vi "Process Collision.vi"(11 "Ball-Goal Post in":refnum<class "Ball-Goal Post.lvclass">) -> (3 "Ball-Goal Post out":refnum<class "Ball-Goal Post.lvclass">)   [LabVIEW 2021, in "Ball-Goal Post.lvclass"]
doc: "MIT Licence\nCopyright (c) 2024 David Grollier"
uses:
  Ball-Goal Post.lvclass
  C:/Users/David/Documents/GameSoccerSpace/Source/Collision/Collision.lvclass
  Game Componants/Game Board Component/Fixed/Board/Goal post/Goal Post.lvclass
  C:/Users/David/Documents/GameSoccerSpace/Source/Game Componants/Game Componants.lvclass
  Collision.lvclass/Collision.ctl
  Game Componants/Game Board Component/Movable/Movable.lvclass/Movable.ctl
  Game Componants/Game Board Component/Fixed/Board/Goal post/Goal Post.lvclass/Goal Post.ctl
  Game Componants/Game Componants.lvclass/Game Componants.ctl
  <vilib>/Analysis/_algsub.llb/Vector Norm.vi
  <vilib>/Analysis/_algsub.llb/Real Vector Norm.vi
  Game Componants/Game Board Component/Movable/Movable.lvclass
  C:/Users/David/Documents/GameSoccerSpace/Source/Game Componants/Game Board Component/Game Board Component.lvclass
  Collision.lvclass
  Game Componants/Game Componants.lvclass
  Utils/Utils.lvlib
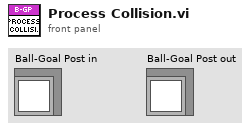
[diagram p1: front panel]
types:
  T1 = typedef "Coordinates.ctl" = cluster{"x":dbl, "y":dbl}
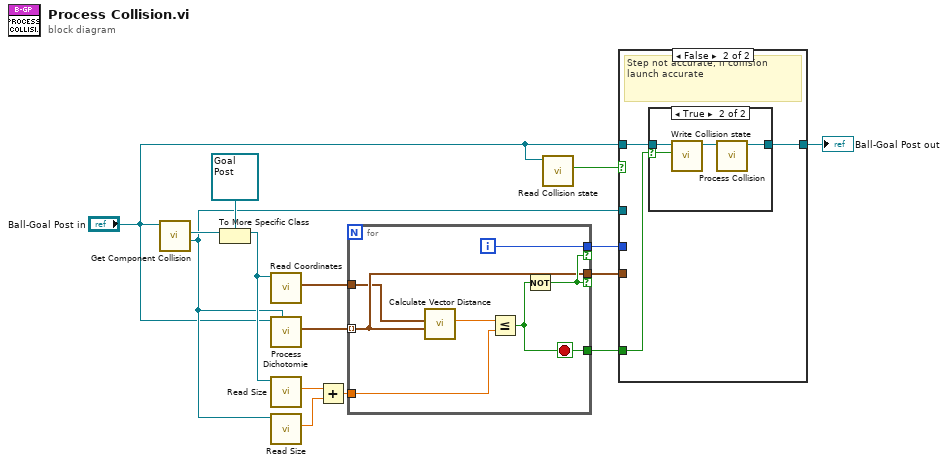
[diagram p0: block diagram]
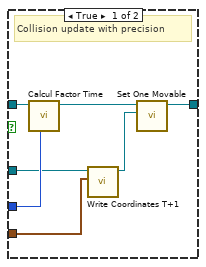
[diagram p2: hidden frame]
diagram:
  n1 = call "Get Component Collision.vi"("Collision in"="Ball-Goal Post in") -> ("Movable out"=w5:refnum<class "Movable.lvclass">, "GB Component out"=w11:refnum<class "Game Board Component.lvclass">)  [unwired: 9 in]
  n2 = To More Specific Class(target class=refnum<class "Goal Post.lvclass"> refnum ("Movable out"), reference=w11) -> (specific class reference=w15:refnum<class "Goal Post.lvclass">)  [unwired: 1 in, 1 out]
  n3 = call "Read Coordinates.vi"("Game Componants in"=w15) -> ("Coordinates"=w8:T1)  [unwired: 10 in]
  n4 = call "Process Dichotomie.vi"("Movable in"=w5, "Collision in"="Ball-Goal Post in") -> ("Coordinates with dichotomie[] out"=w6:T1[])  [unwired: 8 in, 1 out]
  n5 = call "Read Size.vi"("Goal post in"=w15) -> ("Size"=w13:dbl)  [unwired: 10 in]
  n6 = call "Read Size.vi"("Movable in"=w5) -> ("Size"=w12:dbl)  [unwired: 10 in]
  n7 = Add(x=w13, y=w12) -> (x+y=w14:dbl)
  n8 = for {
    tunnel: w14 -> [w22]
    tunnel: w8 -> [w17]
    tunnel: w6 -> [w18] mode=indexing
    tunnel: [w20] -> w1 if=w19
    tunnel: [w18] -> w7 if=w19
    tunnel: [w21] -> w2
    i -> [w20]
    stop <- w21 stop-if-true
    n9 = call "Calculate Vector Distance.vi"("V2"=w18, "V1"=w17) -> ("Distance out"=w16:dbl)  [unwired: 9 in]
    n10 = Less Or Equal?(x=w16, y=w22) -> (x <= y?=w21:bool)
    n11 = Not(x=w21) -> (.not. x?=w19:bool)
  }
  n12 = call "Read Collision state.vi"("Collision in"="Ball-Goal Post in") -> ("Collision state"=w3:bool)  [unwired: 10 in]
  n13 = case shown="False" w3 {
    tunnel: w1 -> [w25 _]
    tunnel: [w28 w31] -> w9
    tunnel: "Ball-Goal Post in" -> [w26 w32]
    tunnel: w5 -> [w23 _]
    tunnel: w7 -> [w27 _]
    tunnel: w2 -> [_ w30]
    frame True {
      # "Collision update with precision"
      n14 = call "Calcul Factor Time.vi"("Accurate Iteration in"=w25, "Collision in"=w26) -> ("Collision out"=w24:refnum<class "Ball-Goal Post.lvclass">)  [unwired: 9 in]
      n15 = call "Write Coordinates T+1.vi"("Coordinates"=w27, "Movable in"=w23) -> ("Movable out"=w29:refnum<class "Movable.lvclass">)  [unwired: 9 in]
      n16 = call "Set One Movable.vi"("Movable in"=w29, "Collision in"=w24) -> ("Collision out"=w28:refnum<class "Ball-Goal Post.lvclass">)  [unwired: 9 in]
    }
    frame False {
      # "Step not accurate, if collision launch accurate"
      n17 = case shown="True" w30 {
        selector: w30 -> [_ w34]
        tunnel: w32 -> [w33 w36]
        tunnel: [w33 w35] -> w31
        frame False {
        }
        frame True {
          n18 = call "Write Collision state.vi"("Collision state"=w34, "Collision in"=w36) -> ("Collision out"=w37:refnum<class "Ball-Goal Post.lvclass">)  [unwired: 9 in]
          n19 = call-dynamic "Process Collision.vi"("Ball-Goal Post in"=w37) -> ("Ball-Goal Post out"=w35:refnum<class "Ball-Goal Post.lvclass">)  [unwired: 10 in]
        }
      }
    }
  }
  "Ball-Goal Post out" <- w9
